vi "AIDI-Clear Tasks.vi"(5 "AI Tasks":T2[](array[typedef]), 9 "DI Tasks":T1) -> (15 "error out":errorcluster)   [LabVIEW 2020]
uses:
  Typedefs/AIDI-Task Specification.ctl
  Typedefs/AIDI-DI Tasks.ctl
  <resource>/objmgr/daqmx.rc
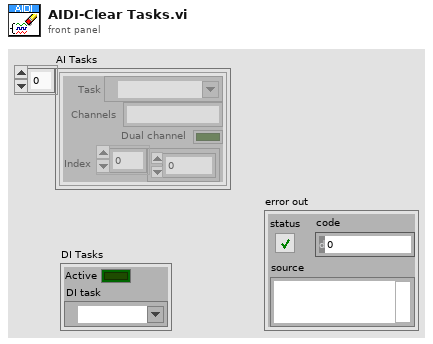
[diagram p1: front panel]
types:
  T1 = typedef "AIDI-DI Tasks.ctl" = cluster{"Active":bool, "DI task":refnum<k21>}
  T2 = typedef "AIDI-Task Specification.ctl" = cluster{"Task":refnum<k21>, "Channels":string, "Dual channel":bool, "Index":i32[]}
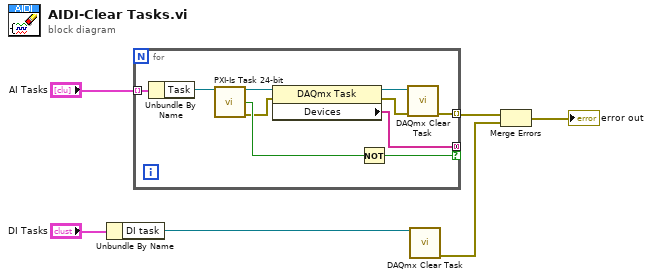
[diagram p0: block diagram]
diagram:
  n1 = Unbundle By Name("DI Tasks") -> ("DI task"=w5:refnum<k21>)
  n2 = for {
    tunnel: "AI Tasks" -> [w16] mode=indexing
    tunnel: [w15] -> w3 mode=indexing
    tunnel: [w11] -> _ mode=concatenating if=w10
    n3 = Unbundle By Name(w16) -> ("Task"=w13:refnum<k21>)
    n4 = call "PXI-Is Task 24-bit.vi"("task"=w13) -> ("task out"=w12:refnum<k21>, "is 24bit?"=w9:bool, "error out"=w8:errorcluster)  [unwired: 9 in, 3 out]
    n5 = property class="DAQmx Task"(reference=w12, error in=w8) -> (reference out=w14:refnum<k21>, error out=w7:errorcluster, "Devices"=w11:tag[])
    n6 = Not(x=w9) -> (.not. x?=w10:bool)
    n7 = call <vilib>:"DAQmx Clear Task.vi"("task in"=w14, "error in"=w7) -> ("error out"=w15:errorcluster)  [unwired: 13 in]
  }
  n8 = call <vilib>:"DAQmx Clear Task.vi"("task in"=w5) -> ("error out"=w2:errorcluster)  [unwired: 14 in]
  n9 = Merge Errors(w3, w2) -> (→"error out":errorcluster)
